vi "Demo test build.vi"() -> ()   [LabVIEW 2014]
panel:
  in  "Boolean":bool
  in  "stop":bool
  out "read buffer":string
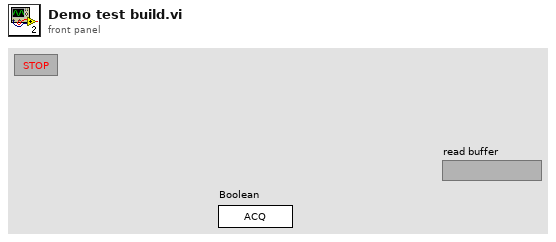
[diagram p1: front panel]
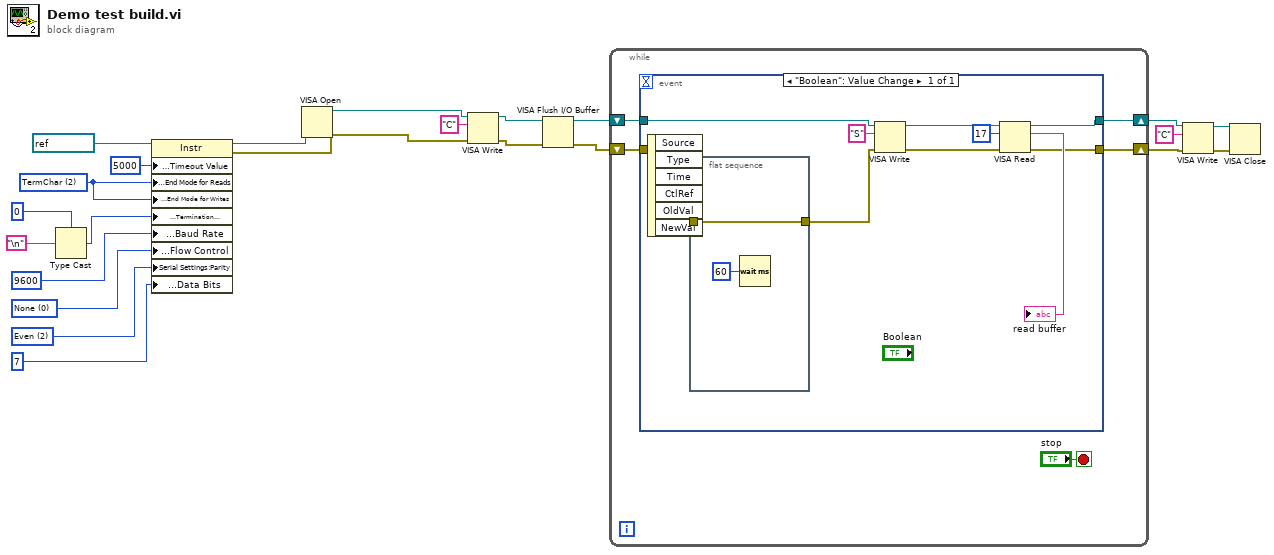
[diagram p0: block diagram]
diagram:
  w15 = u16 2 items=["None", "Odd", "Even", "Mark", "Space"] ("Serial Settings:Parity")
  w16 = u16 0 items=["None", "XON/XOFF", "RTS/CTS", "XON/XOFF & RTS/CTS", "DTR/DSR", "XON/XOFF & DTR/DSR"] ("Serial Settings:Flow Control")
  w18 = u16 2 items=["None", "LastBit", "TermChar"] ("Serial Settings:Serial End Mode for Reads")
  n1 = Type Cast(type=u8 0, x="\n") -> (*(type *) &x=w20:u8)
  n2 = property class="Instr"(reference=refnum<visa-resource-name> "COM6", "General Settings:Timeout Value"=u32 5000, "Serial Settings:End Mode for Reads"=w18, "Serial Settings:End Mode for Writes"=w18, "Message Based Settings:Termination Character"=w20, "Serial Settings:Baud Rate"=u32 9600, "Serial Settings:Flow Control"=w16, "Serial Settings:Parity"=w15, "Serial Settings:Data Bits"=u16 7) -> (reference out=w23:refnum<visa-resource-name>, error out=w24:errorcluster)  [unwired: 1 in]
  n3 = VISA Open(error in (no error)=w24, VISA resource name=w23) -> (VISA resource name=w11:refnum<visa-resource-name>, error out=w10:errorcluster)  [unwired: 3 in]
  n4 = VISA Write(VISA resource name=w11, write buffer="C", error in (no error)=w10) -> (VISA resource name out=w7:refnum<visa-resource-name>, error out=w9:errorcluster)  [unwired: 1 out]
  n5 = VISA Flush I/O Buffer(VISA resource name=w7, error in (no error)=w9) -> (VISA resource name out=w6:refnum<visa-resource-name>, error out=w8:errorcluster)  [unwired: 1 in]
  n6 = while {
    shift-right: [w26] -> w1
    shift-left: w8 -> [w29]
    shift-right: [w27] -> w2
    shift-left: w6 -> [w28]
    stop <- "stop" stop-if-true
    n7 = event shown="[0] \"Boolean\": Value Change" {
      selector: _ -> [_]
      dyn-events: _ -> [_]
      timeout: _ -> [_]
      tunnel: w29 -> [w38]
      tunnel: w28 -> [w37]
      tunnel: [w31] -> w27
      tunnel: [w30] -> w26
      event "Boolean": Value Change {
        n8 = event-data() -> ()  [unwired: 1 in, 6 out]
        n9 = flat-sequence {
          tunnel: w38 -> [w40]
          tunnel: [w40] -> w36
          frame #0 {
            n10 = Wait (ms)(milliseconds to wait=u32 60) -> ()  [unwired: 1 out]
          }
        }
        n11 = VISA Write(VISA resource name=w37, write buffer="S", error in (no error)=w36) -> (VISA resource name out=w35:refnum<visa-resource-name>, error out=w34:errorcluster)  [unwired: 1 out]
        n12 = VISA Read(VISA resource name=w35, byte count=u32 17, error in (no error)=w34) -> (VISA resource name out=w31:refnum<visa-resource-name>, read buffer=→"read buffer":string, error out=w30:errorcluster)  [unwired: 1 out]
      }
    }
  }
  n13 = VISA Write(VISA resource name=w2, write buffer="C", error in (no error)=w1) -> (VISA resource name out=w3:refnum<visa-resource-name>, error out=w4:errorcluster)  [unwired: 1 out]
  n14 = VISA Close(VISA resource name=w3, error in (no error)=w4) -> ()  [unwired: 1 out]
